vi "HP amp control.vi"() -> ()   [LabVIEW 2011]
uses:
  <vilib>/Instr/_visa.llb/VISA Open Access Mode.ctl
panel:
  out "error out":errorcluster
  in  "VISA GPIB Resource":refnum<visa-resource-name>="GPIB0::10::INSTR"
  in  "string to write":string="AM:STAT OFF;:FREQ 12GHZ"
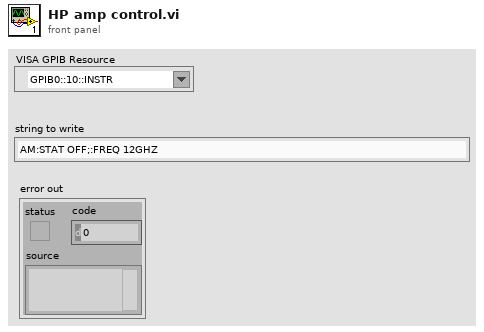
[diagram p1: front panel]
types:
  T1 = typedef "VISA Open Access Mode.ctl" = u32
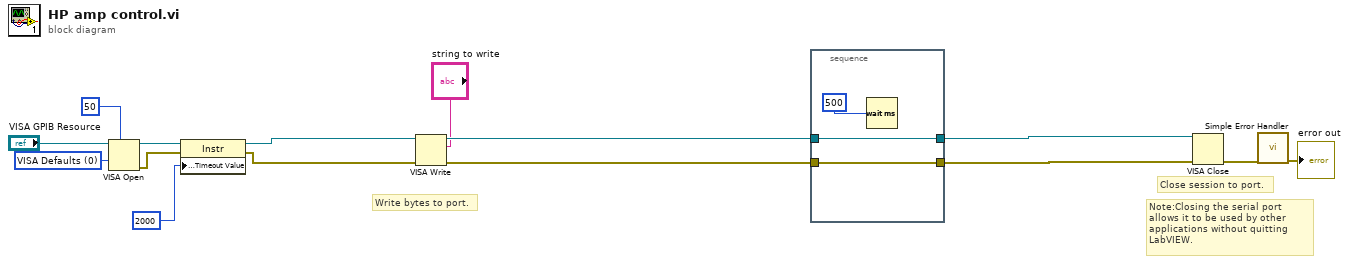
[diagram p0: block diagram]
diagram:
  w4 = T1 0 items=["VISA Defaults"=0, "Exclusive Lock"=1, "Load Configured Settings"=4] ("Access Mode")
  # "Write bytes to port."
  # "Note:Closing the serial port allows it to be used by other applications without quitting LabVIEW."
  # "Close session to port."
  n1 = VISA Open(timeout (0)=u32 50 ("VISA Open timeout (0)"), access mode=w4, VISA resource name="VISA GPIB Resource") -> (VISA resource name=w7:refnum<visa-resource-name>, error out=w6:errorcluster)  [unwired: 2 in]
  n2 = property class="Instr"(reference=w7, error in=w6, "General Settings:Timeout Value"=u32 2000) -> (reference out=w3:refnum<visa-resource-name>, error out=w2:errorcluster)
  n3 = VISA Write(VISA resource name=w3, write buffer="string to write", error in (no error)=w2) -> (VISA resource name out=w13:refnum<visa-resource-name>, error out=w14:errorcluster)  [unwired: 1 out]
  n4 = stacked-sequence {
    tunnel: w14 -> [w18]
    tunnel: [w18] -> w10
    tunnel: w13 -> [w17]
    tunnel: [w17] -> w11
    frame #0 {
      n5 = Wait (ms)(milliseconds to wait=u32 500 ("delay before read (ms)")) -> ()  [unwired: 1 out]
    }
  }
  n6 = VISA Close(VISA resource name=w11, error in (no error)=w10) -> (error out=w15:errorcluster)
  n7 = call <vilib>:"Simple Error Handler.vi"("error in (no error)"=w15) -> ("error out"=→"error out":errorcluster)  [unwired: 1 in, 7 out]
